vi "Main.vi"(8 "error in (no error)":errorcluster, 11 "StageSPIMBase in":refnum<class "StageSPIM.lvclass">) -> (0 "error out":errorcluster, 3 "component":refnum<class "StageSPIM.lvclass">)   [LabVIEW 2012, in "StageSPIM.lvclass"]
doc: "Main VI of the component."
uses:
  StageSPIM.lvclass
  <vilib>/Distrio/Murmex/Murmex/command_enum.ctl
  StageSPIM.lvclass/StageSPIM.ctl
  <vilib>/Distrio/Murmex/InitialiseMessage/InitialiseMessage.lvclass
  <vilib>/Distrio/Murmex/GenericMessage/GenericMessage.lvclass
  <vilib>/Distrio/Murmex/TerminateMessage/TerminateMessage.lvclass
  <vilib>/Distrio/Murmex/Murmex/update_cluster.ctl
  <vilib>/Distrio/Murmex/StopMessage/StopMessage.lvclass
  <vilib>/Distrio/Murmex/ConfigureMessage/ConfigureMessage.lvclass
  <vilib>/Distrio/Murmex/Murmex/Set configure at initialise.vi
  <vilib>/Distrio/Murmex/Murmex/Set log reference.vi
  <vilib>/Distrio/Murmex/Murmex/Set VI reference.vi
  <vilib>/Distrio/Murmex/Murmex/Get ID.vi
  <vilib>/Distrio/Murmex/Murmex/Set write log to disk.vi
  <vilib>/Distrio/Murmex/Murmex/Murmex.lvclass
  <vilib>/Distrio/Murmex/Message/Message.lvclass
panel:
  in  "button::stop":bool
  in  "button::configure":bool
  in  "button::quit":bool
  in  "Tab Control":enum32{"Main", "Debug"}(tab)
  in  "forwardFocus":bool
  in  "backFocus":bool
  in  "stepFocus":dbl[unit]
  out "currentFocus":dbl[unit]
  in  "speedFocus":dbl[unit]
  in  "targetFocus":dbl[unit]
  in  "forwardY":bool
  in  "backY":bool
  in  "stepY":dbl[unit]
  in  "forwardZ":bool
  in  "backZ":bool
  in  "stepZ":dbl[unit]
  in  "forwardX":bool
  in  "backX":bool
  in  "stepX":dbl[unit]
  out "currentX":dbl[unit]
  out "currentY":dbl[unit]
  out "currentZ":dbl[unit]
  in  "speedZ":dbl[unit]
  in  "speedY":dbl[unit]
  in  "speedX":dbl[unit]
  in  "targetX":dbl[unit]
  in  "targetY":dbl[unit]
  in  "targetZ":dbl[unit]
  in  "button::send":bool
  out "log":string
  in  "command":T1
  in  "Generic command":string
  in  "ID":string
  out "terminate?":bool=TRUE
  # "Current\nposition"
  # "Target\nposition"
  # "Steps"
  # "Speed"
  # "X"
  # "Y"
  # "Z"
  # "Focus"
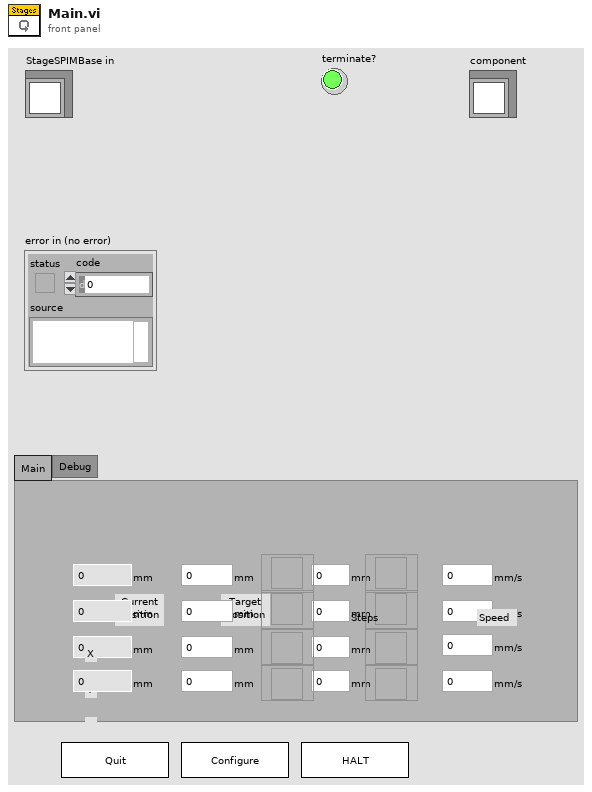
[diagram p1: front panel]
types:
  T1 = typedef "Murmex.lvlib/Murmex.lvclass/command_enum.ctl" = enum16{"null", "initialise", "reset", "terminate", "acknowledge", "update", "inspect", "inform", "proceed", "start", "stop", "fetch", "configure", "generic"}
  T2 = enum8{"Enabled", "Disabled", "Disabled and Grayed Out"}
  T3 = typedef "Murmex.lvlib/Murmex.lvclass/update_cluster.ctl" = cluster{"target ID":string, "key chains":string[], "values":variant[]}
  T4 = typedef "Murmex.lvlib/Murmex.lvclass/Event type enumerations.ctl" = enum16{"before", "after"}
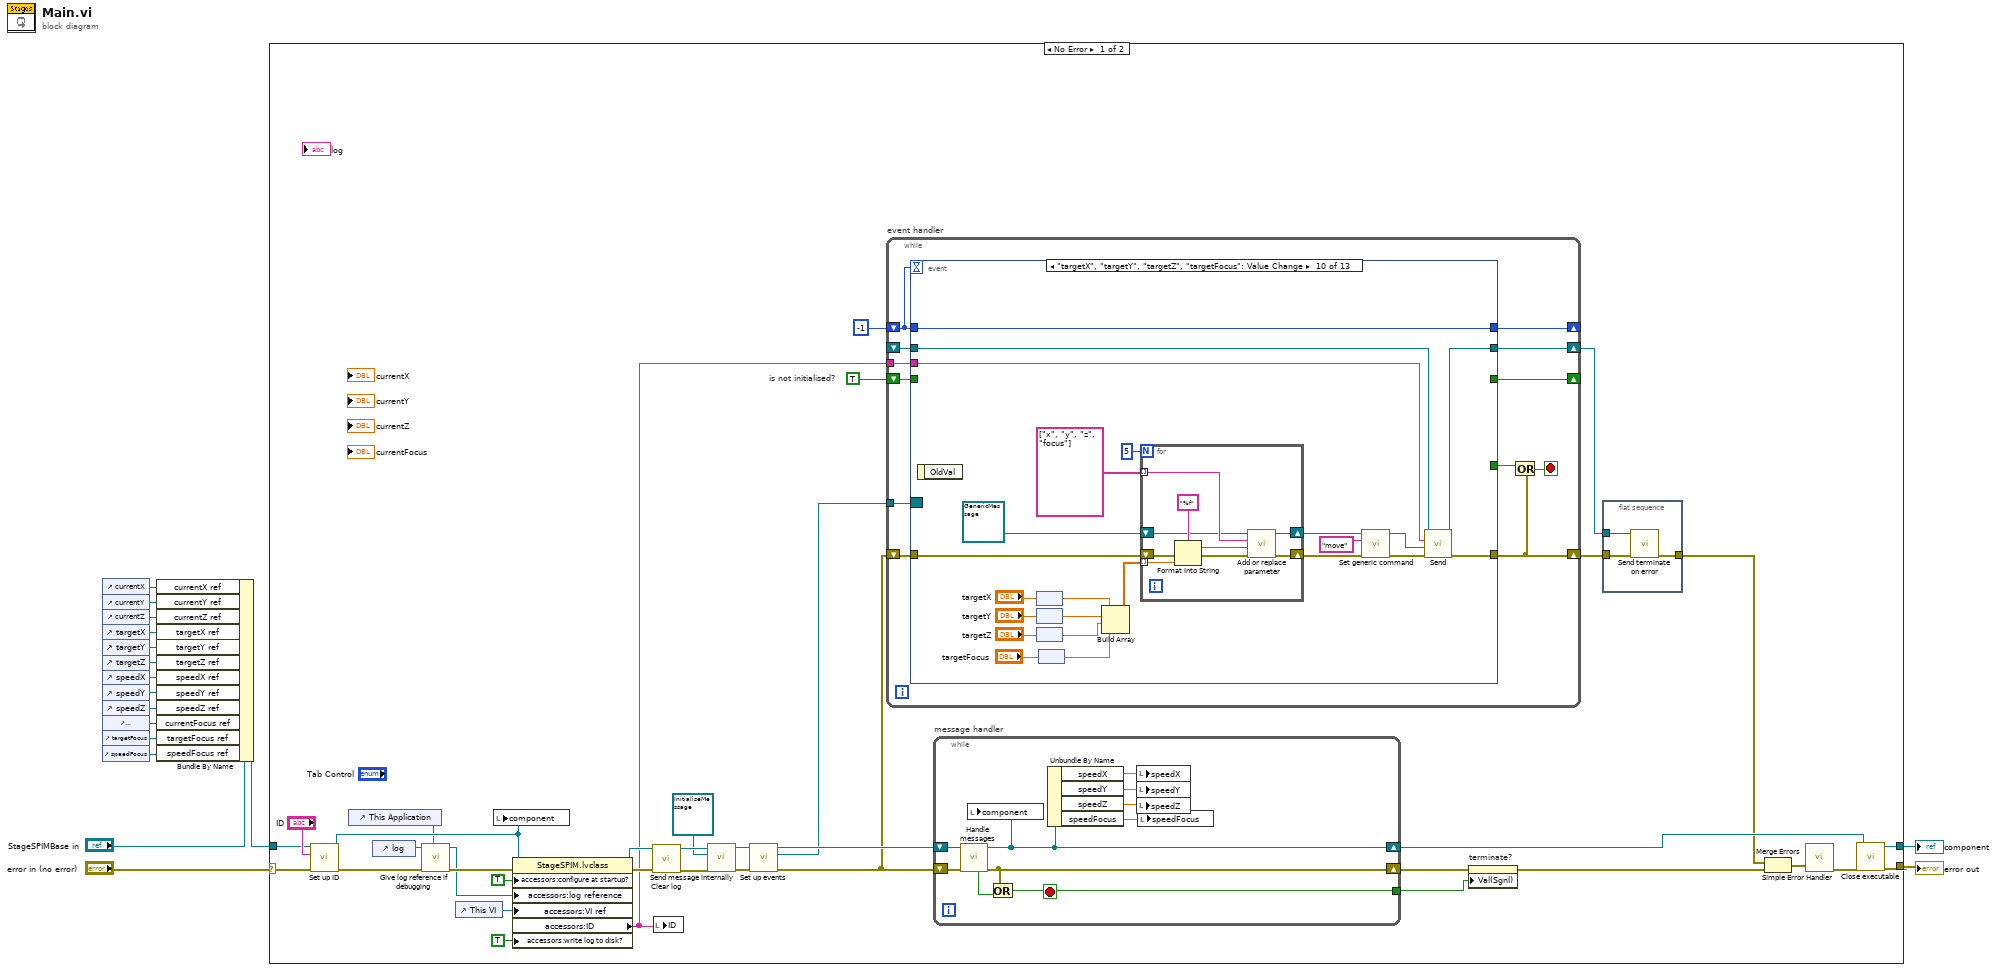
[diagram p0: block diagram]
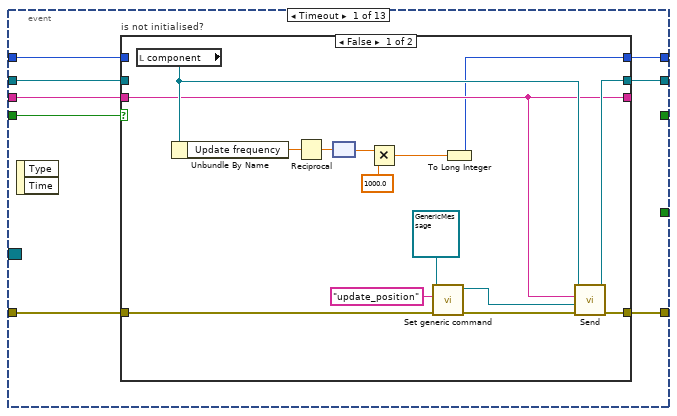
[diagram p2: hidden frame]
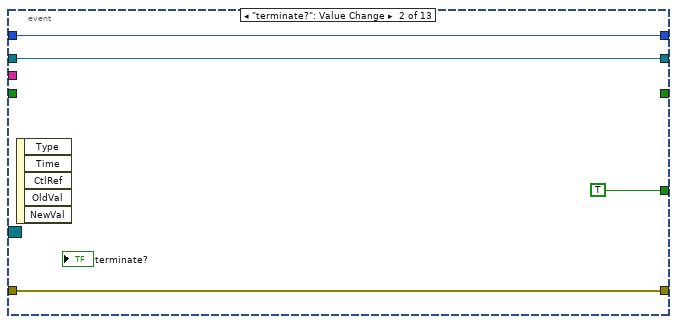
[diagram p4: hidden frame]
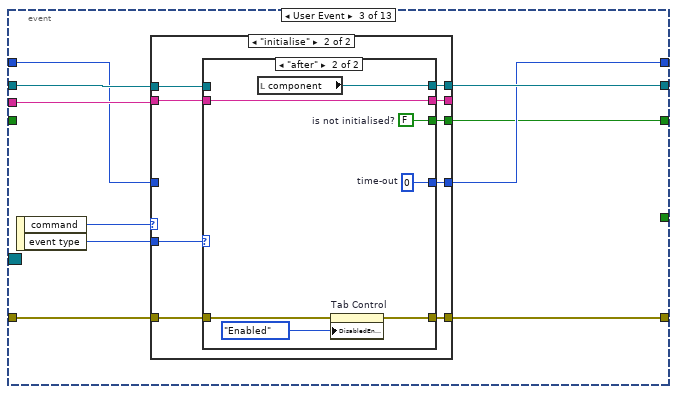
[diagram p5: hidden frame]
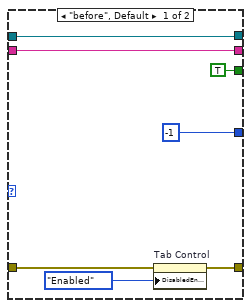
[diagram p7: hidden frame]
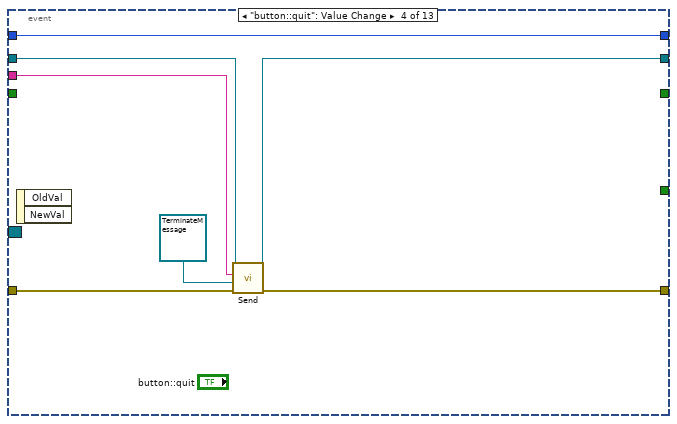
[diagram p8: hidden frame]
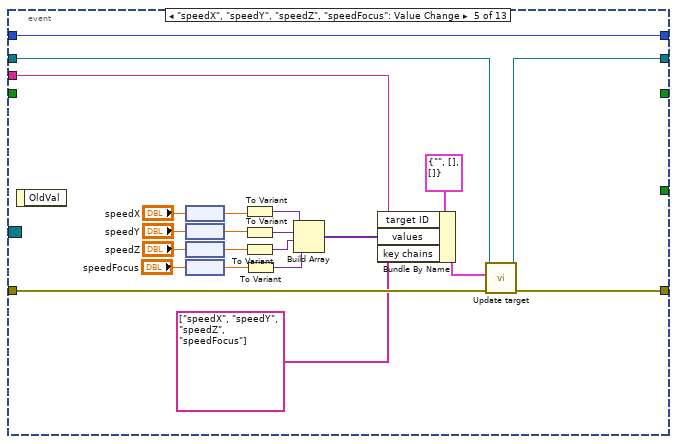
[diagram p9: hidden frame]
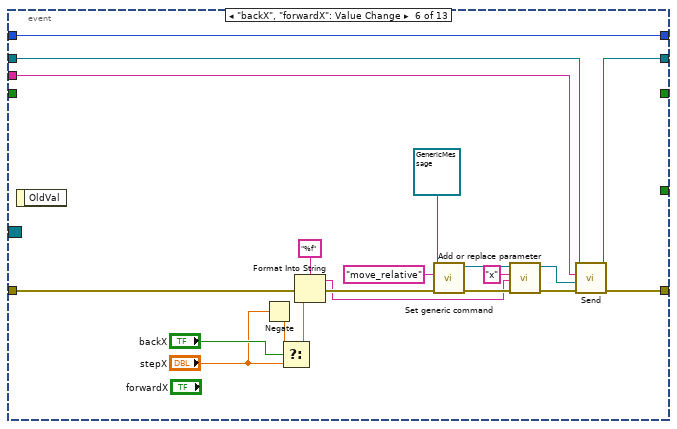
[diagram p10: hidden frame]
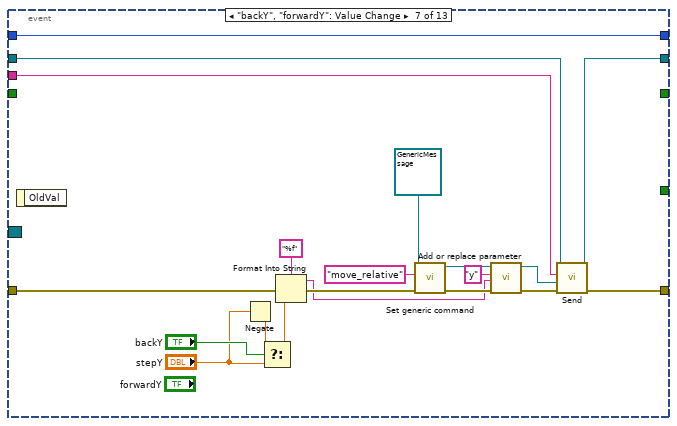
[diagram p11: hidden frame]
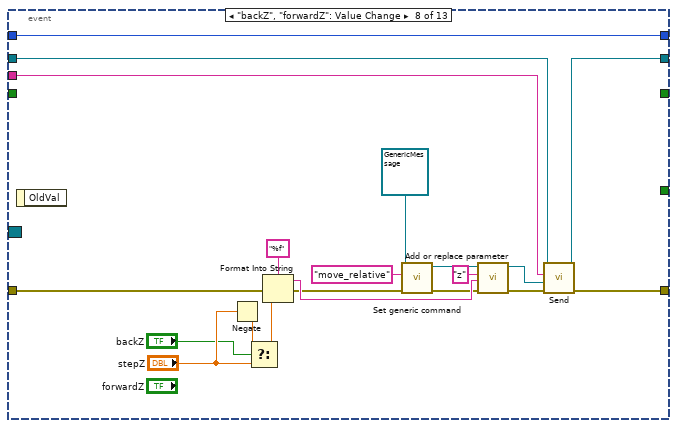
[diagram p12: hidden frame]
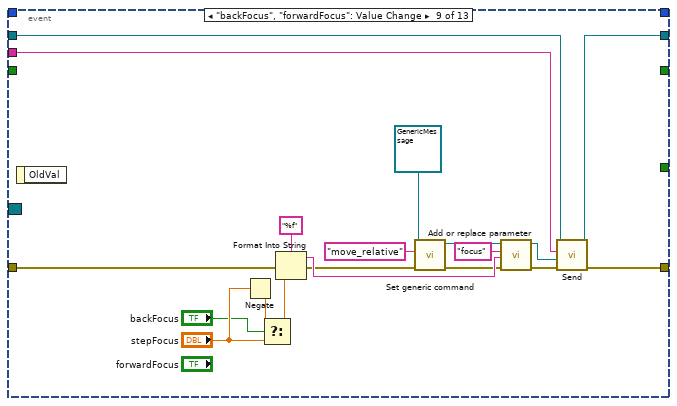
[diagram p13: hidden frame]
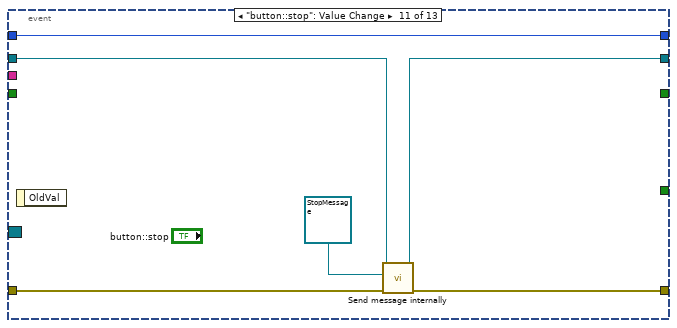
[diagram p14: hidden frame]
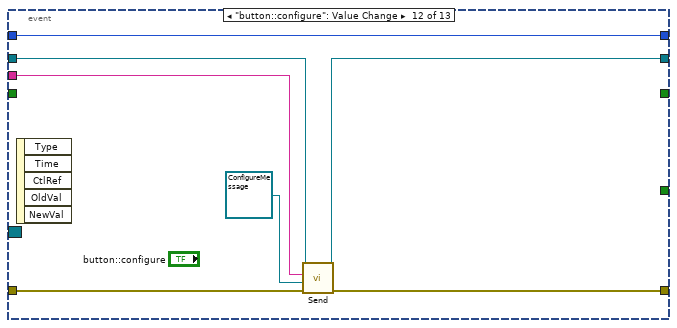
[diagram p15: hidden frame]
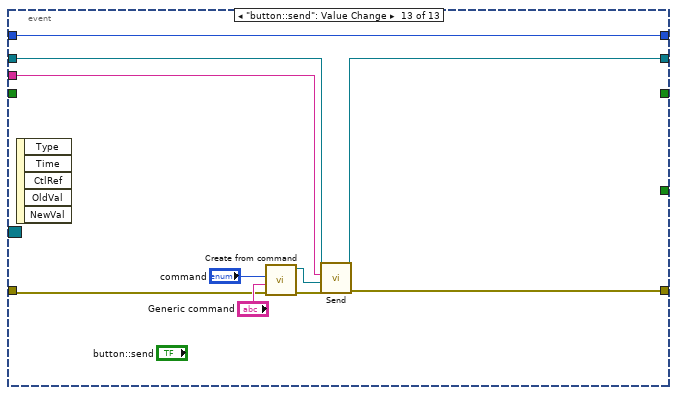
[diagram p16: hidden frame]
diagram:
  n1 = control-ref of="currentX"() -> (w12:refnum<vi>)
  n2 = control-ref of="currentY"() -> (w11:refnum<vi>)
  n3 = control-ref of="currentZ"() -> (w10:refnum<vi>)
  n4 = control-ref of="targetX"() -> (w9:refnum<vi>)
  n5 = control-ref of="targetY"() -> (w8:refnum<vi>)
  n6 = control-ref of="targetZ"() -> (w7:refnum<vi>)
  n7 = control-ref of="speedX"() -> (w6:refnum<vi>)
  n8 = control-ref of="speedY"() -> (w5:refnum<vi>)
  n9 = control-ref of="speedZ"() -> (w4:refnum<vi>)
  n10 = control-ref of="currentFocus"() -> (w3:refnum<vi>)
  n11 = control-ref of="targetFocus"() -> (w2:refnum<vi>)
  n12 = control-ref of="speedFocus"() -> (w1:refnum<vi>)
  n13 = Bundle By Name(cluster="StageSPIMBase in", "currentX ref"=w12, "currentY ref"=w11, "currentZ ref"=w10, "targetX ref"=w9, "targetY ref"=w8, "targetZ ref"=w7, "speedX ref"=w6, "speedY ref"=w5, "speedZ ref"=w4, "currentFocus ref"=w3, "targetFocus ref"=w2, "speedFocus ref"=w1) -> (w15:refnum<class "StageSPIM.lvclass">)
  n14 = case shown="No Error" "error in (no error)" {
    selector: "error in (no error)" -> [w52 w310]
    tunnel: w15 -> [w51 w311]
    tunnel: [w38 w310] -> w14
    tunnel: [w36 w311] -> w13
    frame No Error {
      w28 = TRUE  # is not initialised?
      n15 = call <vilib>:"Set up ID.vi"("error in (no error)"=w52, "component ID"="ID", "MurmexBase in"=w51) -> ("error out"=w23:errorcluster, "MurmexBase out"=w29:refnum<class "StageSPIM.lvclass">)  [unwired: 6 in, 1 out]
      n16 = control-ref of="This Application"() -> (w20:refnum<vi>)
      n17 = control-ref of="log"() -> (w21:refnum<vi>)
      n18 = call "Give log reference if debugging.vi"("application ref"=w20, "error in (no error)"=w23, "log reference in"=w21) -> ("error out"=w22:errorcluster, "log reference out"=w19:refnum<vi>)  [unwired: 6 in, 1 out]
      n19 = control-ref of="This VI"() -> (w49:refnum<vi>)
      n20 = local write "component"(w29) -> ()
      n21 = property class="StageSPIM.lvclass"(reference=w29, error in=w22, "accessors:configure at startup?"=TRUE ("configure at startup?"), "accessors:log reference"=w19, "accessors:VI ref"=w49, "accessors:write log to disk?"=TRUE ("write log to disk?")) -> (reference out=w47:refnum<class "StageSPIM.lvclass">, error out=w48:errorcluster, "accessors:ID"=w30:string)
      n22 = call <vilib>:"Clear log.vi"("error in (no error)"=w48, "MurmexBase in"=w47) -> ("error out"=w46:errorcluster, "MurmexBase out"=w45:refnum<class "StageSPIM.lvclass">)  [unwired: 8 in]
      n23 = local write "ID"(w30) -> ()
      n24 = call <vilib>:"Send message internally.vi"("error in (no error)"=w46, "Message"=refnum<class "InitialiseMessage.lvclass"> refnum ("Distrio Murmex 1.1:InitialiseMessage"), "Murmex in"=w45) -> ("error out"=w43:errorcluster, "Murmex out"=w42:refnum<class "StageSPIM.lvclass">)  [unwired: 7 in]
      n25 = call <vilib>:"Set up events.vi"("error in (no error)"=w43, "MurmexBase in"=w42) -> ("error out"=w35:errorcluster, "Event Registration Refnum"=w34:refnum<event-registration>, "MurmexBase out"=w41:refnum<class "StageSPIM.lvclass">)  [unwired: 7 in]
      n26 = while "event handler" {
        shift-right: [w59] -> w32
        shift-left: w35 -> [w68]
        tunnel: w34 -> [w67]
        shift-right: [w65] -> _
        shift-left: -1 -> [w66]
        shift-right: [w62] -> w24
        shift-left: _ -> [w61]
        shift-right: [w57] -> _
        shift-left: w28 -> [w58]
        tunnel: w30 -> [w63]
        stop <- w64 stop-if-true
        n27 = event shown="[9] \"targetX\", \"targetY\", \"targetZ\", \"targetFocus\": Value Change" {
          selector: w67 -> [_ _ _ _ _ _ _ _ _ _ _ _ _]
          dyn-events: _ -> [_ _ _ _ _ _ _ _ _ _ _ _ _]
          timeout: w66 -> [_ _ _ _ _ _ _ _ _ _ _ _ _]
          tunnel: w68 -> [w75 w99 w109 w142 w164 w167 w189 w209 w229 w248 w282 w289 w295]
          tunnel: w66 -> [w69 w97 w101 w137 w151 w166 w188 w210 _ w262 w280 w283 w291]
          tunnel: [w76 w97 w102 w137 w151 w166 w188 w210 _ w262 w280 w283 w291] -> w65
          tunnel: [w74 w99 w103 w141 w163 w173 w193 w212 w232 w266 w278 w288 w294] -> w59
          tunnel: w63 -> [w73 _ w106 w138 w162 w170 w190 w211 w226 w263 _ w286 w290]
          tunnel: w61 -> [w71 w96 w105 w140 w161 w171 w191 w206 w228 w264 w281 w285 w293]
          tunnel: [w72 w96 w104 w139 w160 w172 w192 w213 w227 w265 w279 w284 w292] -> w62
          tunnel: [_ TRUE _ _ _ _ _ _ _ _ _ _ _] -> w60
          tunnel: w58 -> [w70 _ _ _ _ _ _ _ _ _ _ _ _]
          tunnel: [_ _ w100 _ _ _ _ _ _ _ _ _ _] -> w57
          event Timeout {
            n28 = event-data() -> ()  [unwired: 1 in, 2 out]
            n29 = case "is not initialised?" shown="False" w70 {
              tunnel: [w77 w92] -> w76
              tunnel: w75 -> [w85 w95]
              tunnel: [w84 w95] -> w74
              tunnel: w73 -> [w80 w94]
              tunnel: [w82 w93] -> w72
              tunnel: w71 -> [_ w93]
              tunnel: [w80 w94] -> _
              tunnel: w69 -> [_ w92]
              frame False {
                n30 = local read "component"() -> (w81:refnum<class "StageSPIM.lvclass">)
                n31 = Unbundle By Name(w81) -> ("Update frequency"=w91:dbl[unit])
                n32 = Reciprocal(x=w91) -> (1/x=w90:dbl[unit])
                n33 = node(w90) -> (w79:dbl)
                n34 = Multiply(x=w79, y=1000.0) -> (x*y=w78:dbl)
                n35 = call <vilib>:"Set generic command.vi"("error in (no error)"=w85, "generic command"="update_position", "GenericMessage in"=refnum<class "GenericMessage.lvclass"> refnum ("Distrio Murmex 1.1:GenericMessage")) -> ("error out"=w86:errorcluster, "GenericMessage out"=w83:refnum<class "GenericMessage.lvclass">)  [unwired: 7 in]
                n36 = To Long Integer(number=w78) -> (32bit integer=w77:i32)
                n37 = call <vilib>:"Send.vi"("error in (no error)"=w86, "Message"=w83, "recipient"=w80, "Murmex in"=w81) -> ("error out"=w84:errorcluster, "Murmex out"=w82:refnum<class "StageSPIM.lvclass">)  [unwired: 6 in]
              }
              frame True {
              }
            }
          }
          event "terminate?": Value Change {
            n38 = event-data() -> ()  [unwired: 1 in, 5 out]
          }
          event User Event {
            n39 = event-data() -> ("command"=w108:T1, "event type"=w107:T4)  [unwired: 1 in]
            n40 = case shown="\"initialise\"" w108 {
              tunnel: w109 -> [w111 w122]
              tunnel: [w111 w121] -> w103
              tunnel: w106 -> [w113 w120]
              tunnel: [w112 w119] -> w104
              tunnel: w105 -> [w112 w118]
              tunnel: [w113 w117] -> _
              tunnel: w107 -> [_ w116]
              tunnel: [w110 w115] -> w102
              tunnel: w101 -> [w110 _]
              tunnel: [_ w114] -> w100
              frame "null", Default {
              }
              frame "initialise" {
                n41 = case shown="\"after\"" w116 {
                  tunnel: [w128 w135] -> w121
                  tunnel: w122 -> [w129 w136]
                  tunnel: w120 -> [w126 w132]
                  tunnel: [w125 w134] -> w119
                  tunnel: w118 -> [w125 _]
                  tunnel: [w126 w132] -> w117
                  tunnel: [-1 w131] -> w115
                  tunnel: [TRUE ("is not initialised?") w130] -> w114
                  frame "before", Default {
                    n42 = property on="Tab Control" class="TabCtl (strict)"(error in=w129, "DisabledEnum"=T2."Enabled" ("Disabled")) -> (error out=w128:errorcluster)  [unwired: 1 in, 1 out]
                  }
                  frame "after" {
                    w130 = FALSE  # is not initialised?
                    w131 = 0  # time-out
                    n43 = local read "component"() -> (w134:refnum<class "StageSPIM.lvclass">)
                    n44 = property on="Tab Control" class="TabCtl (strict)"(error in=w136, "DisabledEnum"=T2."Enabled" ("Disabled")) -> (error out=w135:errorcluster)  [unwired: 1 in, 1 out]
                  }
                }
              }
            }
          }
          event "button::quit": Value Change {
            n45 = event-data() -> ()  [unwired: 1 in, 2 out]
            n46 = call <vilib>:"Send.vi"("error in (no error)"=w142, "Message"=refnum<class "TerminateMessage.lvclass"> refnum ("Murmex.lvlib:TerminateMessage"), "recipient"=w138, "Murmex in"=w140) -> ("error out"=w141:errorcluster, "Murmex out"=w139:refnum<class "StageSPIM.lvclass">)  [unwired: 6 in]
          }
          event "speedX", "speedY", "speedZ", "speedFocus": Value Change {
            n47 = event-data() -> ()  [unwired: 1 in, 1 out]
            n48 = node("speedX") -> (w148:dbl)
            n49 = node("speedY") -> (w149:dbl)
            n50 = node("speedZ") -> (w150:dbl)
            n51 = node("speedFocus") -> (w146:dbl)
            n52 = To Variant(anything=w148) -> (Variant=w156:variant)
            n53 = To Variant(anything=w149) -> (Variant=w155:variant)
            n54 = To Variant(anything=w150) -> (Variant=w154:variant)
            n55 = To Variant(anything=w146) -> (Variant=w145:variant)
            n56 = Build Array(w156, w155, w154, w145) -> (w153:variant[])
            n57 = Bundle By Name(cluster=T3 {"target ID"="", "key chains"=[], "values"=[]} ("update cluster"), "target ID"=w162, "values"=w153, "key chains"=string[] ["speedX", "speedY", "speedZ", "speedFocus"]) -> (w144:T3)
            n58 = call <vilib>:"Update target.vi"("error in (no error)"=w164, "update cluster"=w144, "MurmexBase in"=w161) -> ("error out"=w163:errorcluster, "MurmexBase out"=w160:refnum<class "StageSPIM.lvclass">)  [unwired: 7 in]
          }
          event "backX", "forwardX": Value Change {
            n59 = event-data() -> ()  [unwired: 1 in, 1 out]
            n60 = Negate(x="stepX") -> (-x=w180:dbl[unit])
            n61 = Select(t=w180, s="backX", f="stepX") -> (s? t:f=w175:dbl[unit])
            n62 = Format Into String(format string="%f", error in=w167, w175) -> (resulting string=w176:string, error out=w179:errorcluster)  [unwired: 1 in]
            n63 = call <vilib>:"Set generic command.vi"("error in (no error)"=w179, "generic command"="move_relative", "GenericMessage in"=refnum<class "GenericMessage.lvclass"> refnum ("Distrio Murmex 1.1:GenericMessage")) -> ("error out"=w184:errorcluster, "GenericMessage out"=w182:refnum<class "GenericMessage.lvclass">)  [unwired: 7 in]
            n64 = call <vilib>:"Add or replace parameter.vi"("error in (no error)"=w184, "value"=w176, "name"="x", "Message in"=w182) -> ("error out"=w183:errorcluster, "Message out"=w177:refnum<class "GenericMessage.lvclass">)  [unwired: 6 in]
            n65 = call <vilib>:"Send.vi"("error in (no error)"=w183, "Message"=w177, "recipient"=w170, "Murmex in"=w171) -> ("error out"=w173:errorcluster, "Murmex out"=w172:refnum<class "StageSPIM.lvclass">)  [unwired: 6 in]
          }
          event "backY", "forwardY": Value Change {
            n66 = event-data() -> ()  [unwired: 1 in, 1 out]
            n67 = Negate(x="stepY") -> (-x=w200:dbl[unit])
            n68 = Select(t=w200, s="backY", f="stepY") -> (s? t:f=w195:dbl[unit])
            n69 = Format Into String(format string="%f", error in=w189, w195) -> (resulting string=w196:string, error out=w199:errorcluster)  [unwired: 1 in]
            n70 = call <vilib>:"Set generic command.vi"("error in (no error)"=w199, "generic command"="move_relative", "GenericMessage in"=refnum<class "GenericMessage.lvclass"> refnum ("Distrio Murmex 1.1:GenericMessage")) -> ("error out"=w204:errorcluster, "GenericMessage out"=w202:refnum<class "GenericMessage.lvclass">)  [unwired: 7 in]
            n71 = call <vilib>:"Add or replace parameter.vi"("error in (no error)"=w204, "value"=w196, "name"="y", "Message in"=w202) -> ("error out"=w203:errorcluster, "Message out"=w197:refnum<class "GenericMessage.lvclass">)  [unwired: 6 in]
            n72 = call <vilib>:"Send.vi"("error in (no error)"=w203, "Message"=w197, "recipient"=w190, "Murmex in"=w191) -> ("error out"=w193:errorcluster, "Murmex out"=w192:refnum<class "StageSPIM.lvclass">)  [unwired: 6 in]
          }
          event "backZ", "forwardZ": Value Change {
            n73 = event-data() -> ()  [unwired: 1 in, 1 out]
            n74 = Negate(x="stepZ") -> (-x=w219:dbl[unit])
            n75 = Select(t=w219, s="backZ", f="stepZ") -> (s? t:f=w224:dbl[unit])
            n76 = Format Into String(format string="%f", error in=w209, w224) -> (resulting string=w223:string, error out=w220:errorcluster)  [unwired: 1 in]
            n77 = call <vilib>:"Set generic command.vi"("error in (no error)"=w220, "generic command"="move_relative", "GenericMessage in"=refnum<class "GenericMessage.lvclass"> refnum ("Distrio Murmex 1.1:GenericMessage")) -> ("error out"=w215:errorcluster, "GenericMessage out"=w217:refnum<class "GenericMessage.lvclass">)  [unwired: 7 in]
            n78 = call <vilib>:"Add or replace parameter.vi"("error in (no error)"=w215, "value"=w223, "name"="z", "Message in"=w217) -> ("error out"=w216:errorcluster, "Message out"=w222:refnum<class "GenericMessage.lvclass">)  [unwired: 6 in]
            n79 = call <vilib>:"Send.vi"("error in (no error)"=w216, "Message"=w222, "recipient"=w211, "Murmex in"=w206) -> ("error out"=w212:errorcluster, "Murmex out"=w213:refnum<class "StageSPIM.lvclass">)  [unwired: 6 in]
          }
          event "backFocus", "forwardFocus": Value Change {
            n80 = event-data() -> ()  [unwired: 1 in, 1 out]
            n81 = Negate(x="stepFocus") -> (-x=w238:dbl[unit])
            n82 = Select(t=w238, s="backFocus", f="stepFocus") -> (s? t:f=w243:dbl[unit])
            n83 = Format Into String(format string="%f", error in=w229, w243) -> (resulting string=w242:string, error out=w239:errorcluster)  [unwired: 1 in]
            n84 = call <vilib>:"Set generic command.vi"("error in (no error)"=w239, "generic command"="move_relative", "GenericMessage in"=refnum<class "GenericMessage.lvclass"> refnum ("Distrio Murmex 1.1:GenericMessage")) -> ("error out"=w234:errorcluster, "GenericMessage out"=w236:refnum<class "GenericMessage.lvclass">)  [unwired: 7 in]
            n85 = call <vilib>:"Add or replace parameter.vi"("error in (no error)"=w234, "value"=w242, "name"="focus", "Message in"=w236) -> ("error out"=w235:errorcluster, "Message out"=w241:refnum<class "GenericMessage.lvclass">)  [unwired: 6 in]
            n86 = call <vilib>:"Send.vi"("error in (no error)"=w235, "Message"=w241, "recipient"=w226, "Murmex in"=w228) -> ("error out"=w232:errorcluster, "Murmex out"=w227:refnum<class "StageSPIM.lvclass">)  [unwired: 6 in]
          }
          event "targetX", "targetY", "targetZ", "targetFocus": Value Change {
            n87 = event-data() -> ()  [unwired: 1 in, 1 out]
            n88 = node("targetX") -> (w253:dbl)
            n89 = node("targetY") -> (w250:dbl)
            n90 = node("targetZ") -> (w247:dbl)
            n91 = node("targetFocus") -> (w245:dbl)
            n92 = Build Array(w253, w250, w247, w245) -> (w249:dbl[])
            n93 = for {
              N: 5 -> [_]
              shift-right: [w274] -> w259
              shift-left: w248 -> [w273]
              tunnel: string[] ["x", "y", "z", "focus"] -> [w272] mode=indexing
              shift-right: [w270] -> w255
              shift-left: refnum<class "GenericMessage.lvclass"> refnum ("Distrio Murmex 1.1:GenericMessage") -> [w271]
              tunnel: w249 -> [w269] mode=indexing
              n94 = Format Into String(format string="%f", error in=w273, w269) -> (resulting string=w268:string, error out=w275:errorcluster)  [unwired: 1 in]
              n95 = call <vilib>:"Add or replace parameter.vi"("error in (no error)"=w275, "value"=w268, "name"=w272, "Message in"=w271) -> ("error out"=w274:errorcluster, "Message out"=w270:refnum<class "GenericMessage.lvclass">)  [unwired: 6 in]
            }
            n96 = call <vilib>:"Set generic command.vi"("error in (no error)"=w259, "generic command"="move", "GenericMessage in"=w255) -> ("error out"=w261:errorcluster, "GenericMessage out"=w260:refnum<class "GenericMessage.lvclass">)  [unwired: 7 in]
            n97 = call <vilib>:"Send.vi"("error in (no error)"=w261, "Message"=w260, "recipient"=w263, "Murmex in"=w264) -> ("error out"=w266:errorcluster, "Murmex out"=w265:refnum<class "StageSPIM.lvclass">)  [unwired: 6 in]
          }
          event "button::stop": Value Change {
            n98 = event-data() -> ()  [unwired: 1 in, 1 out]
            n99 = call <vilib>:"Send message internally.vi"("error in (no error)"=w282, "Message"=refnum<class "StopMessage.lvclass"> refnum ("Distrio Murmex 1.5:StopMessage"), "Murmex in"=w281) -> ("error out"=w278:errorcluster, "Murmex out"=w279:refnum<class "StageSPIM.lvclass">)  [unwired: 7 in]
          }
          event "button::configure": Value Change {
            n100 = event-data() -> ()  [unwired: 1 in, 5 out]
            n101 = call <vilib>:"Send.vi"("error in (no error)"=w289, "Message"=refnum<class "ConfigureMessage.lvclass"> refnum ("Distrio Murmex 1.1:ConfigureMessage"), "recipient"=w286, "Murmex in"=w285) -> ("error out"=w288:errorcluster, "Murmex out"=w284:refnum<class "StageSPIM.lvclass">)  [unwired: 6 in]
          }
          event "button::send": Value Change {
            n102 = event-data() -> ()  [unwired: 1 in, 5 out]
            n103 = call <vilib>:"Create from command.vi"("error in (no error)"=w295, "generic command"="Generic command", "command"="command") -> ("error out"=w297:errorcluster, "Message out"=w298:refnum<class "Message.lvclass">)  [unwired: 7 in]
            n104 = call <vilib>:"Send.vi"("error in (no error)"=w297, "Message"=w298, "recipient"=w290, "Murmex in"=w293) -> ("error out"=w294:errorcluster, "Murmex out"=w292:refnum<class "StageSPIM.lvclass">)  [unwired: 6 in]
          }
        }
        n105 = Or(x=w60, y=w59) -> (x .or. y?=w64:bool)
      }
      n106 = while "message handler" {
        shift-right: [w307] -> w27
        shift-left: w35 -> [w309]
        shift-right: [w304] -> w37
        shift-left: w41 -> [w308]
        tunnel: [w305] -> w25
        stop <- w305 stop-if-true
        n107 = call <vilib>:"Handle messages.vi"("error in (no error)"=w309, "Murmex in"=w308) -> ("error out"=w307:errorcluster, "Murmex out"=w304:refnum<class "StageSPIM.lvclass">, "terminated?"=w306:bool)  [unwired: 7 in]
        n108 = local write "component"(w304) -> ()
        n109 = Or(x=w307, y=w306) -> (x .or. y?=w305:bool)
        n110 = Unbundle By Name(w304) -> ("speedX"=w303:dbl[unit], "speedY"=w302:dbl[unit], "speedZ"=w301:dbl[unit], "speedFocus"=w300:dbl[unit])
        n111 = local write "speedX"(w303) -> ()
        n112 = local write "speedY"(w302) -> ()
        n113 = local write "speedZ"(w301) -> ()
        n114 = local write "speedFocus"(w300) -> ()
      }
      n115 = property on="terminate?" class="Bool (strict)"(error in=w27, "Val(Sgnl)"=w25) -> (error out=w26:errorcluster)  [unwired: 1 in, 1 out]
      n116 = flat-sequence {
        tunnel: w32 -> [w56]
        tunnel: [w55] -> w31
        tunnel: w24 -> [w54]
        frame #0 {
          n117 = call <vilib>:"Send terminate on error.vi"("error in (no error)"=w56, "Murmex in"=w54) -> ("error out"=w55:errorcluster)  [unwired: 8 in, 1 out]
        }
      }
      n118 = Merge Errors(w31, w26) -> (w40:errorcluster)
      n119 = call <vilib>:"Simple Error Handler.vi"("error in (no error)"=w40) -> ("error out"=w39:errorcluster)  [unwired: 4 in, 4 out]
      n120 = call <vilib>:"Close executable.vi"("error in (no error)"=w39, "MurmexBase in"=w37) -> ("error out"=w38:errorcluster, "MurmexBase out"=w36:refnum<class "StageSPIM.lvclass">)  [unwired: 8 in]
    }
    frame Error {
    }
  }
  "error out" <- w14
  "component" <- w13
